vi "Draw Horizontal Line.vi"(4 "Alpha":dbl, 6 "Colour":u32(colorbox), 7 "Method":T1, 8 "Enable Alpha Blending (F)":bool, 9 "Point 2":T2, 10 "Point 1":T2, 11 "Pixel Data in":u32[][](array[numeric])) -> (3 "Pixel Data out":u32[][](array[numeric]))   [LabVIEW 2020, in "Raster (FPGA).lvlib"]
uses:
  Raster (FPGA).lvlib
  Point 2D (I32).ctl
  Method.ctl
  Global 1.vi
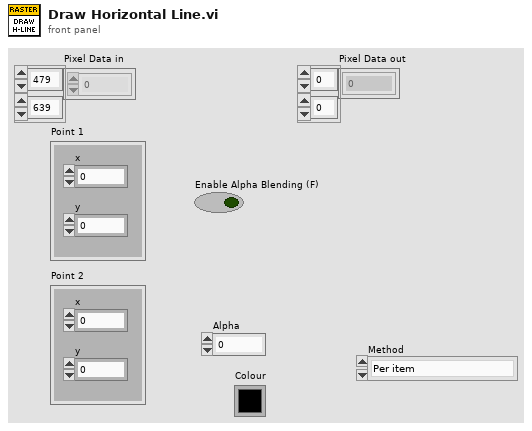
[diagram p1: front panel]
types:
  T1 = typedef "Raster (FPGA).lvlib/Method.ctl" = enum16{"Per item", "Row", "Replace Array Subset", "MoveBlock", " MoveBlock2 "}
  T2 = typedef "Raster (FPGA).lvlib/Point 2D (I32).ctl" = cluster{"x":i32, "y":i32}
  T3 = cluster{"pointer":u64, "size_0":u32, "stride_0":i32, "size_1":u32, "stride_1":i32, "element size":u32, "subarray?":bool}
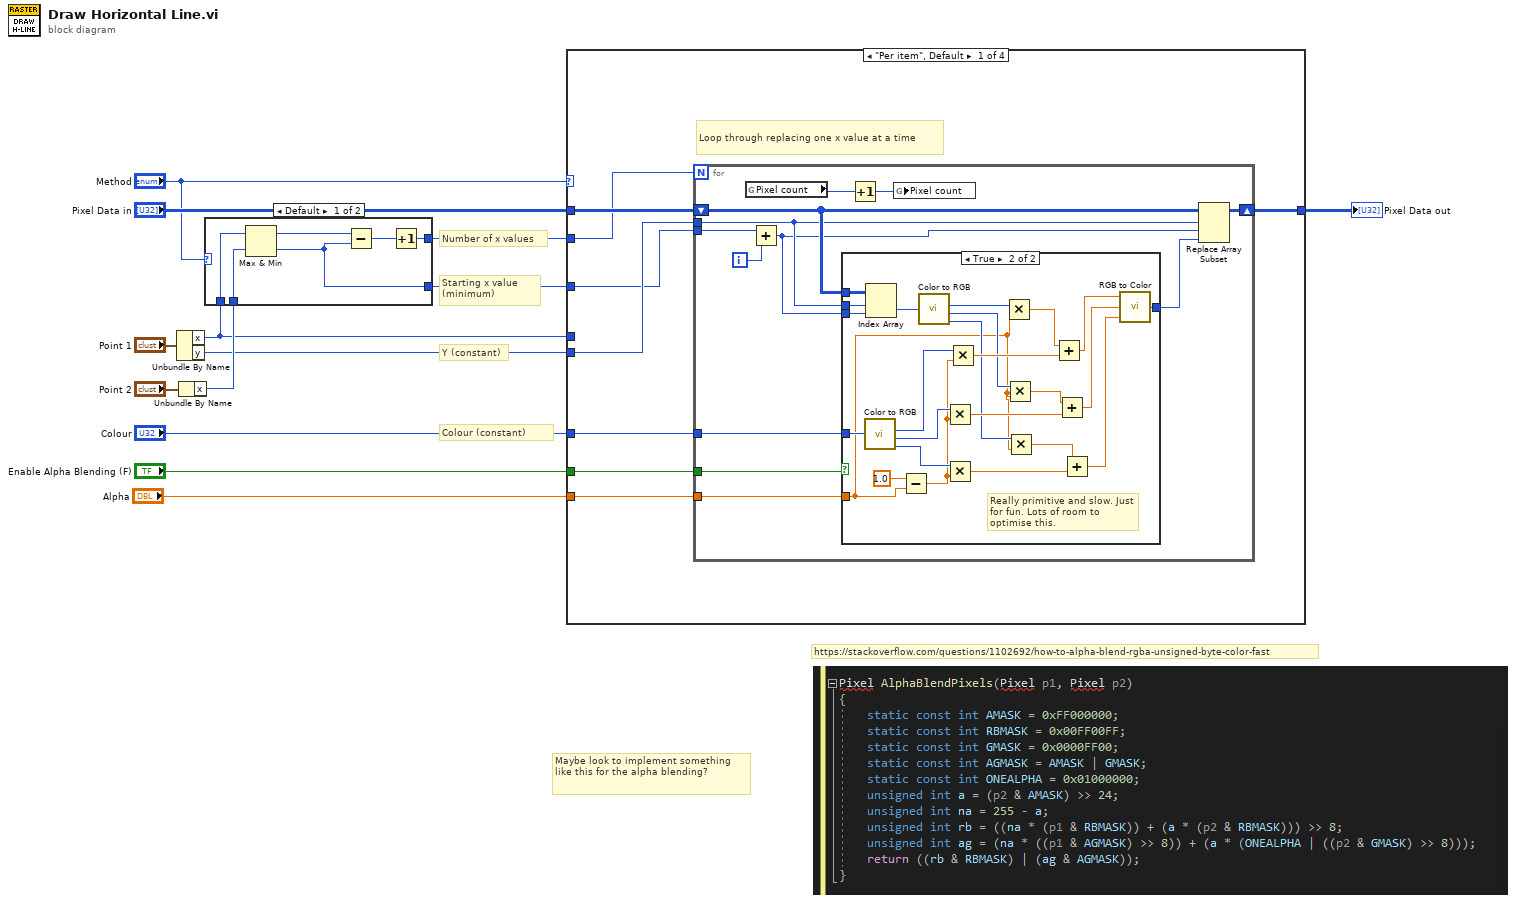
[diagram p0: block diagram]
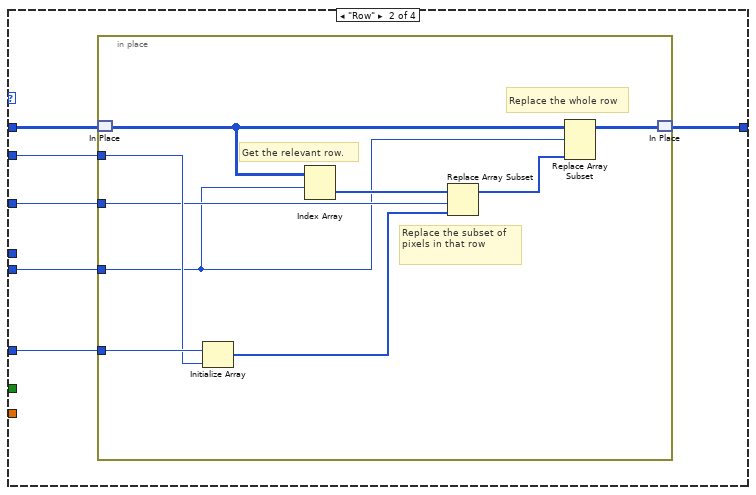
[diagram p4: hidden frame]
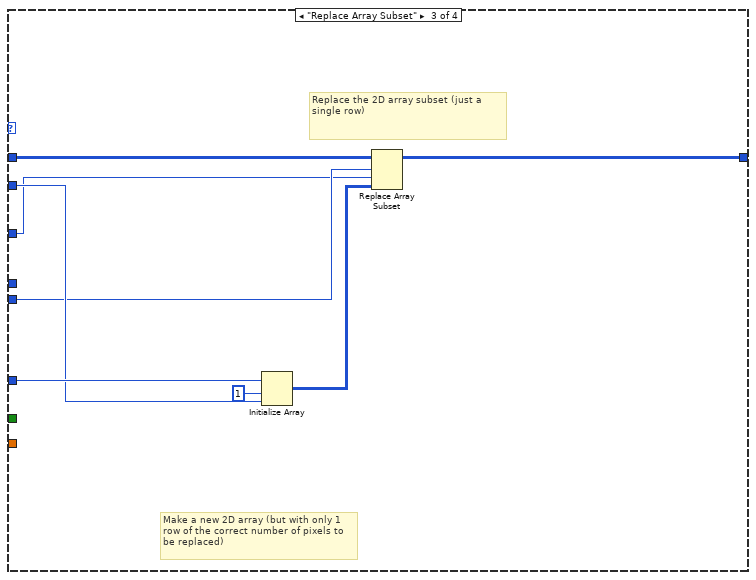
[diagram p5: hidden frame]
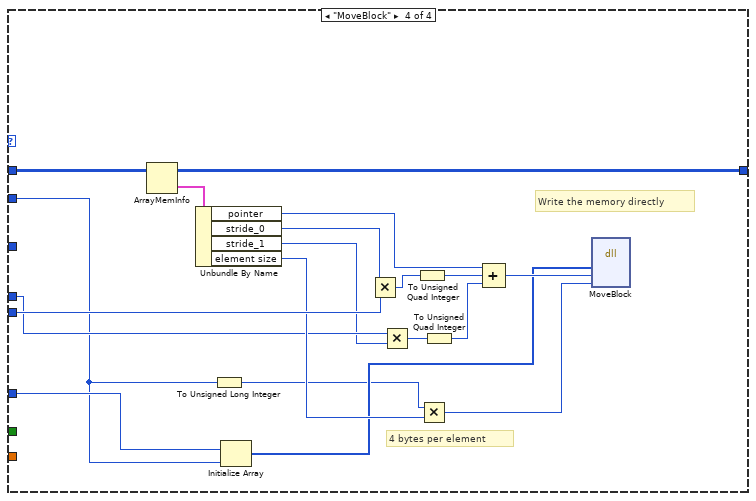
[diagram p6: hidden frame]
diagram:
  # "Maybe look to implement something like this for the alpha blending?"
  # "https://stackoverflow.com/questions/1102692/how-to-alpha-blend-rgba-unsigned-byte-color-fast"
  # "Starting x value\n(minimum)"
  # "Number of x values"
  # "Colour (constant)"
  # "Y (constant)"
  n1 = Unbundle By Name("Point 1") -> ("x"=w4:i32, "y"=w8:i32)
  n2 = Unbundle By Name("Point 2") -> ("x"=w11:i32)
  n3 = case shown="Default" "Method" {
    tunnel: w11 -> [w18 w20]
    tunnel: [w16 w21] -> w9
    tunnel: [w15 w20] -> w7
    tunnel: w4 -> [w14 w21]
    frame Default {
      n4 = Max & Min(x=w14, y=w18) -> (max(x,y)=w17:i32, min(x,y)=w15:i32)
      n5 = Subtract(x=w17, y=w15) -> (x-y=w19:i32)
      n6 = Increment(x=w19) -> (x+1=w16:i32)
    }
    frame " MoveBlock2 " {
    }
  }
  n7 = case shown="\"Per item\", Default" "Method" {
    tunnel: "Pixel Data in" -> [w29 w72 w86 w103]
    tunnel: w9 -> [w28 w71 w84 w90]
    tunnel: w8 -> [w27 w70 w83 w100]
    tunnel: w7 -> [w26 w69 w82 _]
    tunnel: "Colour" -> [w25 w68 w87 w101]
    tunnel: [w24 w67 w85 w102] -> w5
    tunnel: w4 -> [_ _ _ w98]
    tunnel: "Enable Alpha Blending (F)" -> [w23 _ _ _]
    tunnel: "Alpha" -> [w22 _ _ _]
    frame "Per item", Default {
      # "Loop through replacing one x value at a time"
      n8 = for {
        N: w28 -> [_]
        tunnel: w26 -> [w40]
        tunnel: w27 -> [w37]
        shift-right: [w41] -> w24
        shift-left: w29 -> [w38]
        tunnel: w25 -> [w34]
        tunnel: w23 -> [w33]
        tunnel: w22 -> [w32]
        i -> [w39]
        n9 = global read "Global 1.vi" "Pixel count"() -> (w31:u32)
        n10 = Add(x=w40, y=w39) -> (x+y=w36:i32)
        n11 = case shown="True" w33 {
          tunnel: w38 -> [_ w66]
          tunnel: w37 -> [_ w65]
          tunnel: w36 -> [_ w64]
          tunnel: [w42 w63] -> w35
          tunnel: w34 -> [w42 w62]
          tunnel: w32 -> [_ w46]
          frame False {
          }
          frame True {
            # "Really primitive and slow. Just for fun. Lots of room to optimise this."
            n12 = call <vilib>:"Color to RGB.vi"("Color"=w62) -> ("R"=w60:u8, "G"=w59:u8, "B"=w58:u8)  [unwired: 1 out]
            n13 = Index Array(array=w66, index (row)=w65, index (col)=w64) -> (element=w61:u32)
            n14 = Subtract(x=1.0, y=w46) -> (x-y=w47:dbl)
            n15 = call <vilib>:"Color to RGB.vi"("Color"=w61) -> ("R"=w50:u8, "G"=w49:u8, "B"=w48:u8)  [unwired: 1 out]
            n16 = Multiply(x=w59, y=w47) -> (x*y=w55:dbl)
            n17 = Multiply(x=w58, y=w47) -> (x*y=w52:dbl)
            n18 = Multiply(x=w60, y=w47) -> (x*y=w57:dbl)
            n19 = Multiply(x=w50, y=w46) -> (x*y=w45:dbl)
            n20 = Multiply(x=w49, y=w46) -> (x*y=w44:dbl)
            n21 = Multiply(x=w48, y=w46) -> (x*y=w43:dbl)
            n22 = Add(x=w45, y=w57) -> (x+y=w56:dbl)
            n23 = Add(x=w44, y=w55) -> (x+y=w54:dbl)
            n24 = Add(x=w43, y=w52) -> (x+y=w53:dbl)
            n25 = call <vilib>:"RGB to Color.vi"("B"=w53, "G"=w54, "R"=w56) -> ("Color"=w63:u32)
          }
        }
        n26 = Increment(x=w31) -> (x+1=w30:u32)
        n27 = global write "Global 1.vi" "Pixel count"(w30) -> ()
        n28 = Replace Array Subset(array=w38, new element=w35, index (row)=w37, index (col)=w36) -> (w41:u32[][])
      }
    }
    frame "Row" {
      n29 = in-place {
        in-place-border: w68 -> [w81]
        in-place-border: w71 -> [w80]
        in-place-border: w69 -> [w77]
        in-place-border: w70 -> [w76]
        # "Replace the whole row"
        # "Replace the subset of pixels in that row"
        # "Get the relevant row."
        n30 = in-place-match #1(w72) -> (w74:u32[][])
        n31 = Initialize Array(w81, w80) -> (w78:u32[])
        n32 = Index Array(array=w74, index (row)=w76) -> (element=w79:u32[])  [unwired: 1 in]
        n33 = Replace Array Subset(array=w79, new element=w78, index=w77) -> (w75:u32[])
        n34 = Replace Array Subset(array=w74, new element=w75, index (row)=w76) -> (w73:u32[][])  [unwired: 1 in]
        n35 = in-place-match #1(w73) -> (w67:u32[][])
      }
    }
    frame "Replace Array Subset" {
      # "Replace the 2D array subset (just a single row)"
      # "Make a new 2D array (but with only 1 row of the correct number of pixels to be replaced)"
      n36 = Initialize Array(w87, 1 ("dimension size"), w84) -> (w88:u32[][])
      n37 = Replace Array Subset(array=w86, new element=w88, index (row)=w83, index (col)=w82) -> (w85:u32[][])
    }
    frame "MoveBlock" {
      # "Write the memory directly"
      # "4 bytes per element"
      n38 = ArrayMemInfo(3:w103) -> (0:w107:T3, 1:w102:u32[][])
      n39 = Unbundle By Name(w107) -> ("pointer"=w108:u64, "stride_0"=w105:i32, "stride_1"=w97:i32, "element size"=w99:u32)
      n40 = To Unsigned Long Integer(number=w90) -> (unsigned 32bit integer=w91:u32)
      n41 = Initialize Array(w101, w90) -> (w96:u32[])
      n42 = Multiply(x=w105, y=w100) -> (x*y=w93:i32)
      n43 = Multiply(x=w98, y=w97) -> (x*y=w95:i32)
      n44 = To Unsigned Quad Integer(1:w93) -> (0:w92:u64)
      n45 = Multiply(x=w91, y=w99) -> (x*y=w106:u32)
      n46 = To Unsigned Quad Integer(1:w95) -> (0:w94:u64)
      n47 = Compound Arithmetic op=ADD(w108, w92, w94) -> (w104:u64)
      n48 = dll-call lib="LabVIEW" fn="MoveBlock"("Src"=w96, "Dst"=w104, "Size"=w106) -> ()  [unwired: 7 in, 2 out]
    }
  }
  "Pixel Data out" <- w5
